vi "读串口.vi"(0 "VISA resource name":refnum<visa-resource-name>="COM1" caption="VISA资源名称", 1 "baud rate":u32=9600 caption="波特率", 2 "data bits":u16=8 caption="数据比特" min=5 max=8 step=1, 3 "parity":u16(ring) caption="奇偶" items=["无", "奇", "偶", "标记", "空格"], 4 "stop bits":u16(ring)=10 caption="停止位" items=["1.0"=10, "1.5"=15, "2.0"=20], 7 "flow control":u16(ring) caption="流程控制" items=["无"=0, "XON/XOFF"=1, "RTS/CTS"=2, "DTR/DSR"=4]) -> (8 "read string 2":string caption="读取角度", 9 "read string":string caption="读取扭矩", 10 "bytes read":u32 caption="读取的字节")   [LabVIEW 2011]
doc: "基本串口读取和写入范例可实现串口读取、串口写入或者串口读写操作。用户可在前面板选择操作（读取或写入）。如果选择全部，VI将写入数据并读取数据，然后关闭开放给端口的VISA会话句柄。该VI将等待直到端口接收到指定的字节数。\n\n操作步骤：\n1) 选择串行资源并配置参数（波特率、数据位、奇偶、停止位和流控制）。\n2) 选择需执行的操作。\n3) 连接串口至设备。如未发现可用设备，请按以下任一方式执行环回测试。在RS-232线缆中短路引脚2和3，或者在RS-485/422线缆中短路引脚4和8以及引脚5和9。\n4) 运行VI并查看读取的数据。（如果已执行环回测试，“读取字符串”将匹配“写入字符串”。）\n\n注：串口的参数组必须匹配连接仪器或设备的参数。在本范例中，待读取字节参数可指定串口读取的字节数。如端口字节超过指定的字节数，超出部分将不会被读取。如果指定读取的字节数超过实际字节数，可能返回超时错误。\n\n在程序框图中，“配置串口VI”可用于设置配置参数。前面板显示的控件可用于配置基本参数，如波特率、数据位和奇偶。常量可配置其它用户无需设置的参数。“VISA配置串口VI”打开VISA句柄并配置端口后，该VI会将VISA资源名称传递至其它VI以便执行相关操作。“VISA写入”函数将发送一个命令至串行设备，“VISA读取”函数将返回基于该命令的数据。“VISA关闭”函数可关闭该串行设备的引用。关闭引用十分重要，否则可能导致VISA无法通过端口和协议进行通信。"
uses:
  <vilib>/Instr/_visa.llb/VISA Configure Serial Port (Instr).vi
panel:
  in  "delay before read (ms)":u32=2000 caption="读取前延时(ms)"
  # "Windows/Linux用户可使用仪器驱动查找器（帮助>>查找仪器驱动程序）为仪器查找相应的驱动程序。"
  # "选择串口资源以及执行的操作（读取、写入或读写）。如果选择全部，VI将写入数据并读取数据，然后关闭开放给端口的VISA会话句柄。该VI将等待直到端口接收到指定的字节数或者接收到终止符。"
  # "更多信息请选择文件>>VI属性>>说明信息"
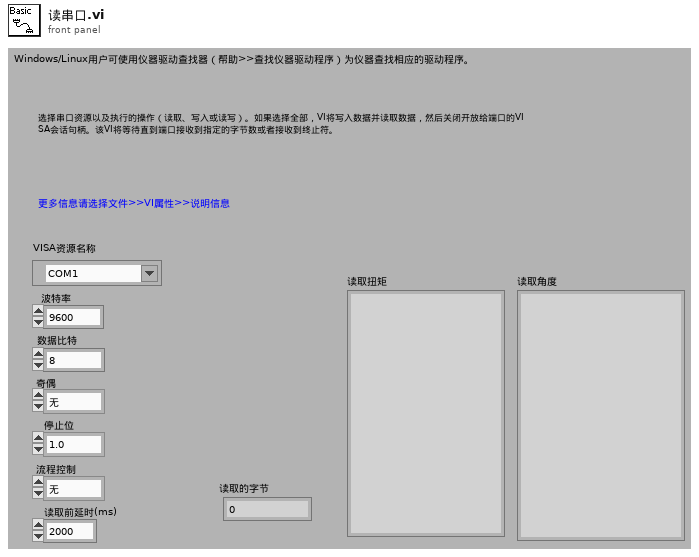
[diagram p1: front panel]
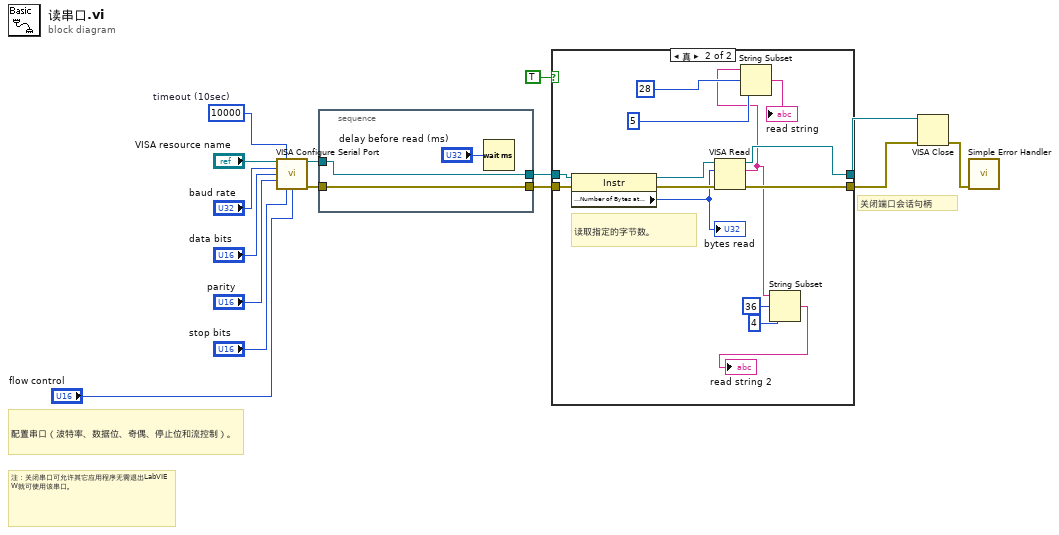
[diagram p0: block diagram]
diagram:
  w9 = u32 10000  # timeout (10sec)
  # "注：关闭串口可允许其它应用程序无需退出LabVIEW就可使用该串口。"
  # "配置串口（波特率、数据位、奇偶、停止位和流控制）。"
  # "关闭端口会话句柄"
  n1 = call-poly "VISA Configure Serial Port"("VISA resource name"="VISA resource name", "timeout (10sec)"=w9, "baud rate (9600)"="baud rate", "data bits (8)"="data bits", "parity (0:none)"="parity", "stop bits (10: 1 bit)"="stop bits", "flow control (0:none)"="flow control") -> ("VISA resource name out"=w3:refnum<visa-resource-name>, "error out"=w2:errorcluster)  [unwired: 2 in, 5 out]
  n2 = stacked-sequence {
    tunnel: w2 -> [w18]
    tunnel: [w18] -> w5
    tunnel: w3 -> [w17]
    tunnel: [w17] -> w4
    frame #0 {
      n3 = Wait (ms)(milliseconds to wait="delay before read (ms)") -> ()  [unwired: 1 out]
    }
  }
  n4 = case shown="真" TRUE {
    tunnel: w5 -> [w20 w30]
    tunnel: [w20 w34] -> w13
    tunnel: [w19 w33] -> w12
    tunnel: w4 -> [w19 w32]
    frame False {
    }
    frame True {
      # "读取指定的字节数。"
      n5 = property class="Instr"(reference=w32, error in=w30) -> (reference out=w31:refnum<visa-resource-name>, error out=w29:errorcluster, "Serial Settings:Number of Bytes at Serial Port"=w28:u32)
      "bytes read" <- w28
      n6 = VISA Read(VISA resource name=w31, byte count=w28, error in (no error)=w29) -> (VISA resource name out=w33:refnum<visa-resource-name>, read buffer=w24:string, error out=w34:errorcluster)  [unwired: 1 out]
      n7 = String Subset(string=w24, offset (0)=28 ("偏移量(0)"), length (rest)=5 ("长度（剩余）")) -> (substring=→"read string":string)
      n8 = String Subset(string=w24, offset (0)=36 ("偏移量(0)"), length (rest)=4 ("长度（剩余）")) -> (substring=→"read string 2":string)
    }
  }
  n9 = VISA Close(VISA resource name=w12, error in (no error)=w13) -> (error out=w11:errorcluster)
  n10 = call <vilib>:"Simple Error Handler.vi"("error in (no error)"=w11) -> ()  [unwired: 1 in, 8 out]
